vi "Teleop-2022-comp.vi"(10 "Match Info":T1={"Autonomous Elapsed Seconds"=0.0, "TeleOp Elapsed Seconds"=0.0, "Disabled Elapsed Seconds"=0.0, "Visited Autonomous"=FALSE, "Visited TeleOp"=FALSE, "Visited Disabled"=FALSE, "Autonomous Settings"={"Autonomous Style"=enum."Independent", "VI Refnum"=refnum}}, 11 "Call Context":T2) -> ()   [LabVIEW 2020]
doc: "This VI is called for each TeleOp packet received from the DS where the robot is not disabled. It is often used to read from the joysticks and update I/O or to update setpoints for timed control loops. It should complete and return within 20 milliseconds or it may miss DS packets."
uses:
  <vilib>/Rock Robotics/WPI/DriverStation/WPI_DriverStationDerivedRobotMode.ctl
  <vilib>/Rock Robotics/WPI/DriverStation/WPI_DriverStationMatch Info.ctl
  <vilib>/Rock Robotics/WPI/Joystick/XBox Buttons Indexer.ctl
  <vilib>/Rock Robotics/WPI/Joystick/XBox Axes Indexer.ctl
  <vilib>/Rock Robotics/WPI/Relay/WPI_RelayValue.ctl
  <vilib>/Rock Robotics/Network Tables/NT Read Boolean.vi
  <vilib>/Rock Robotics/Network Tables/NT Read Number.vi
  Auxilary/AuxGlobals.vi
  Climb/ClimbGlobals.vi
  <vilib>/Rock Robotics/Network Tables/NT Write String.vi
  Human/HumanGlobal.vi
  DriveSystem/DriveGlobals.vi
  <vilib>/Rock Robotics/Network Tables/NT Write Number.vi
  <vilib>/Rock Robotics/Network Tables/NT Write Boolean.vi
  Vision/VisionGlobals.vi
  <vilib>/Rock Robotics/WPI/Joystick/WPI_JoystickArcadeMapping.vi
  <vilib>/Rock Robotics/WPI/ThirdParty/JAS_Junk/TrajLib/Trajectory_Library.lvlib
panel:
  out "Sample Slider 0":dbl(slide) scale=0.0..5.0
  out "Sample Boolean 1":bool
  out "Sample Boolean 0":bool
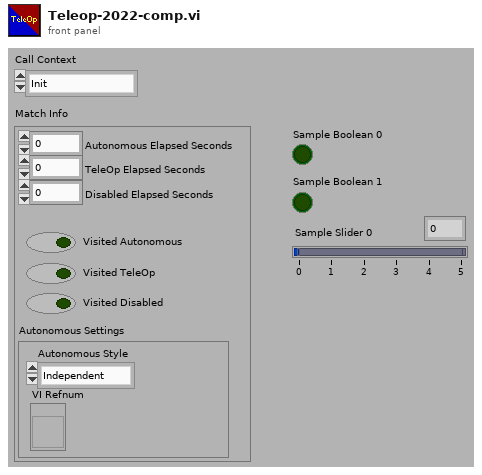
[diagram p1: front panel]
types:
  T1 = typedef "WPI_DriverStationMatch Info.ctl" = cluster{"Autonomous Elapsed Seconds":dbl, "TeleOp Elapsed Seconds":dbl, "Disabled Elapsed Seconds":dbl, "Visited Autonomous":bool, "Visited TeleOp":bool, "Visited Disabled":bool, "Autonomous Settings":cluster{"Autonomous Style":enum16{"Iterative", "Independent"}, "VI Refnum":refnum<vi>}}
  T2 = typedef "WPI_DriverStationDerivedRobotMode.ctl" = enum16{"Init", "Execute", "Stop"}
  T3 = typedef "XBox Buttons Indexer.ctl" = enum16{"A", "B", "X", "Y", "Left Bumper", "Right Bumper", "Back", "Start", "Left Joystick", "Right Joystick"}
  T4 = typedef "XBox Axes Indexer.ctl" = enum16{"Left X", "Left Y", "Left Trigger", "Right Trigger", "Right X", "Right Y"}
  T5 = typedef "WPI_RelayValue.ctl" = enum16{"Off", "On", "Forward", "Reverse"}
  T6 = typedef "WPI_RelayDevRef.ctl" = cluster{"DevStatus":errorcluster, "Relay Channel":T7, "Relay Direction":T8}
  T7 = typedef "FPGA_DIORelayChannel.ctl" = enum8{"Relay 0", "Relay 1", "Relay 2", "Relay 3", "Invalid"}
  T8 = typedef "WPI_RelayDirection.ctl" = enum16{"Both directions", "Forward only", "Reverse only"}
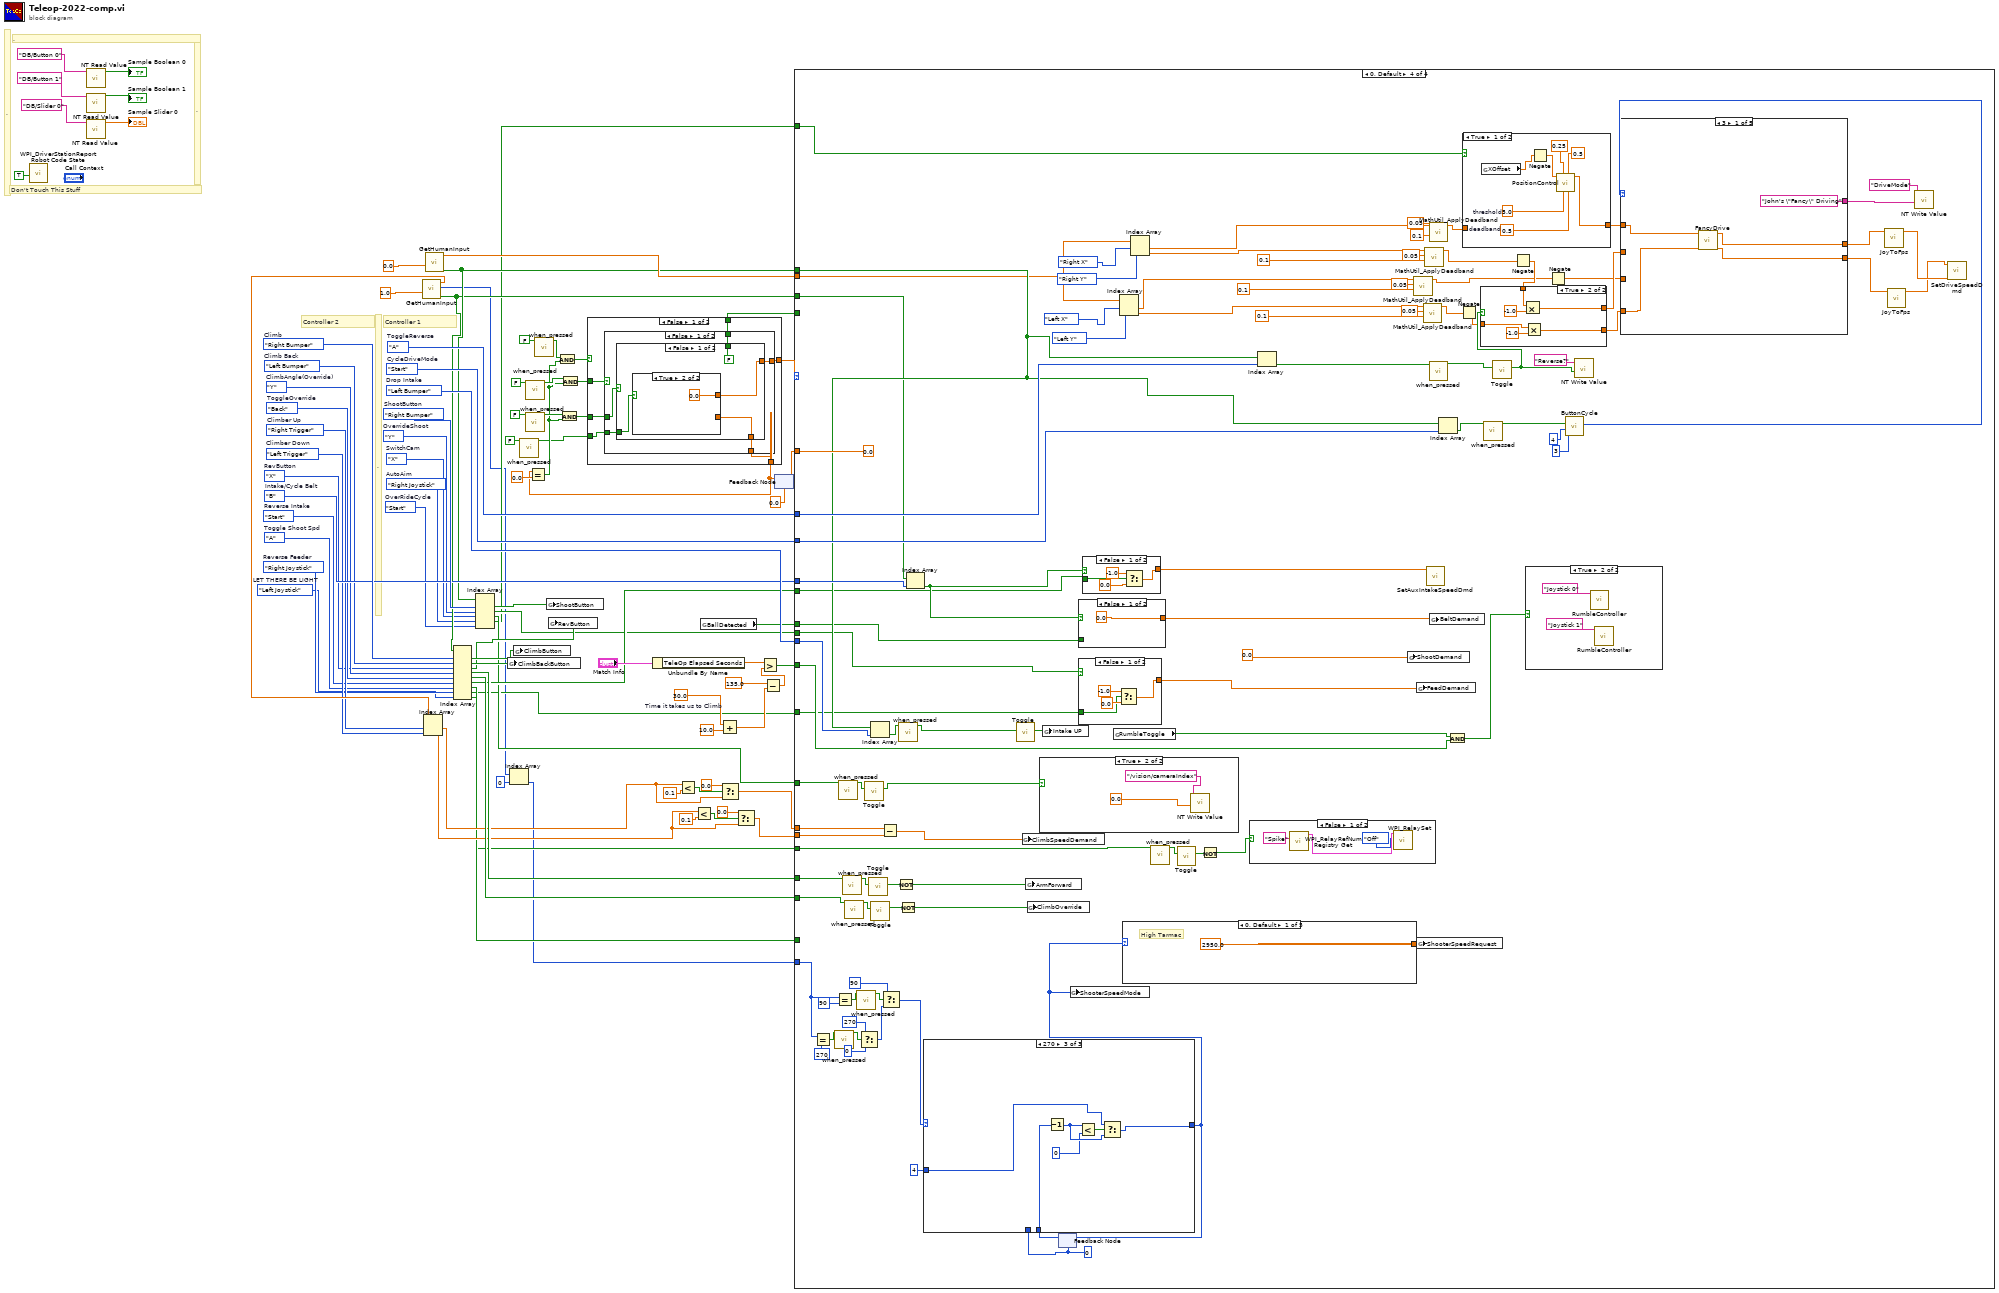
[diagram p0: block diagram]
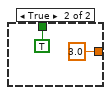
[diagram p3: hidden frame]
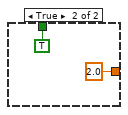
[diagram p4: hidden frame]
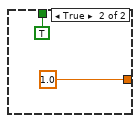
[diagram p5: hidden frame]
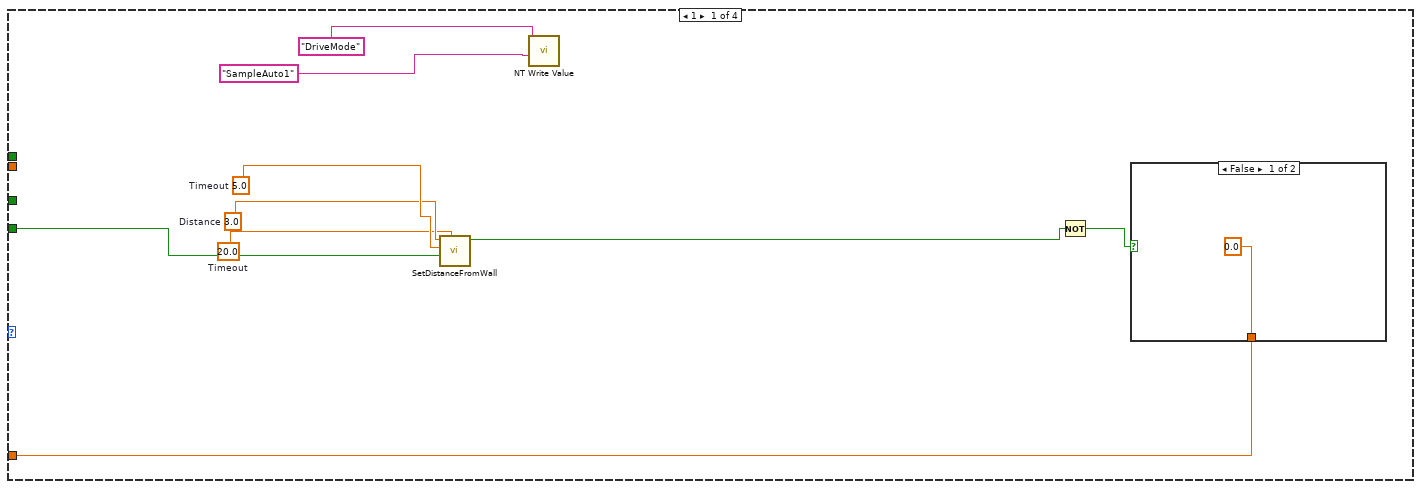
[diagram p6: hidden frame]
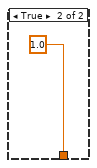
[diagram p7: hidden frame]
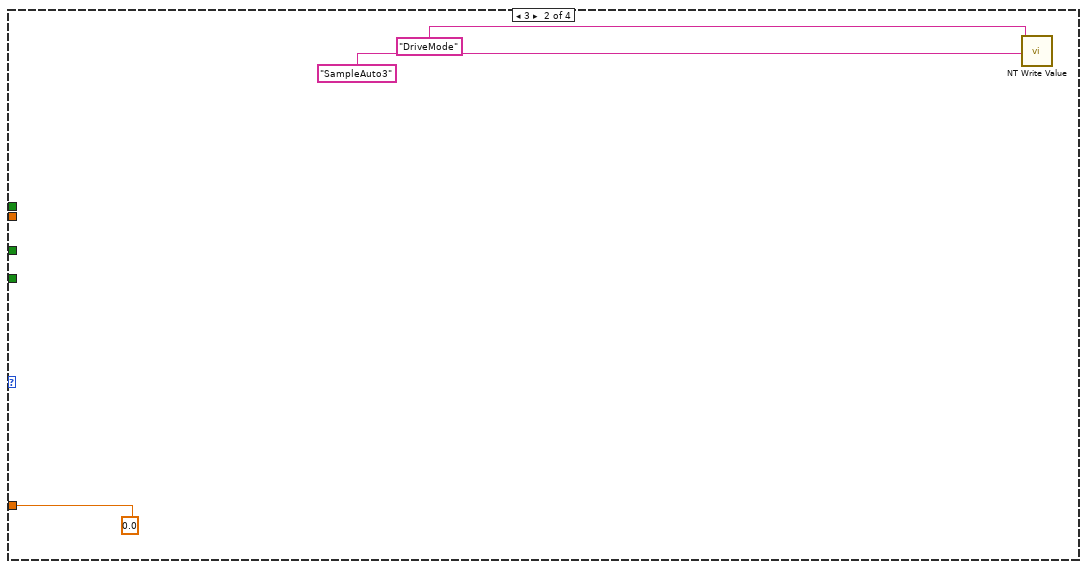
[diagram p8: hidden frame]
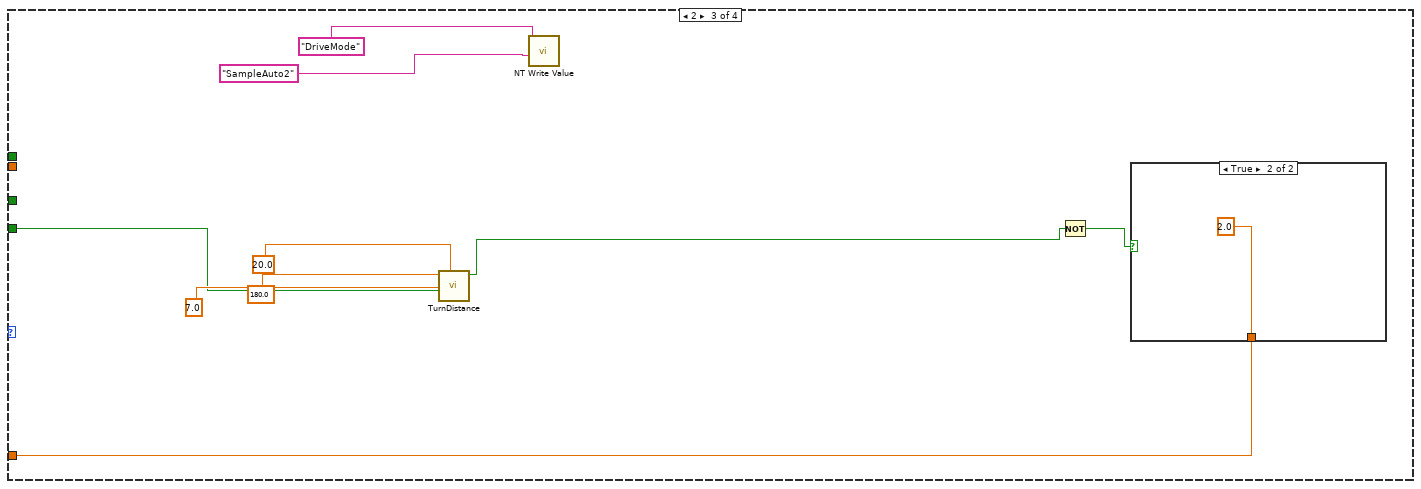
[diagram p9: hidden frame]
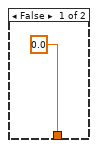
[diagram p10: hidden frame]
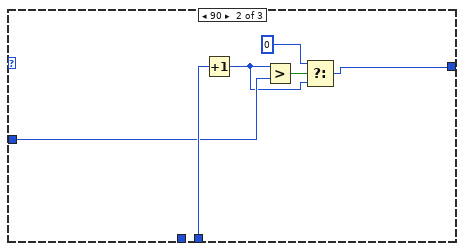
[diagram p12: hidden frame]
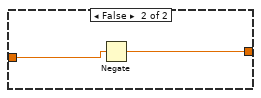
[diagram p13: hidden frame]
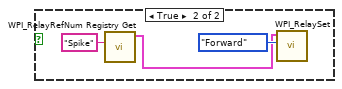
[diagram p14: hidden frame]
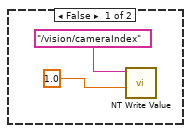
[diagram p15: hidden frame]
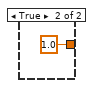
[diagram p16: hidden frame]
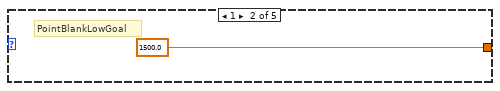
[diagram p17: hidden frame]
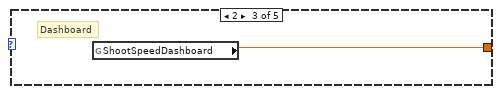
[diagram p18: hidden frame]
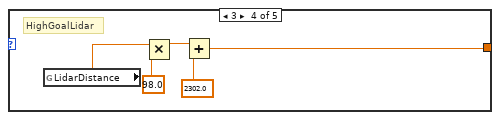
[diagram p19: hidden frame]
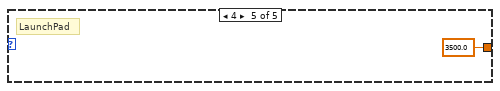
[diagram p20: hidden frame]
diagram:
  w1 = XBox_Buttons_Indexer."Start"  # OverRideCycle
  w6 = XBox_Buttons_Indexer."Right Joystick"  # AutoAim
  w8 = XBox_Buttons_Indexer."Left Joystick"  # LET THERE BE LIGHT
  w10 = XBox_Buttons_Indexer."Right Joystick"  # Reverse Feeder
  w12 = XBox_Buttons_Indexer."X"  # SwitchCam
  w15 = XBox_Buttons_Indexer."Y"  # OverrideShoot
  w17 = XBox_Buttons_Indexer."A"  # Toggle Shoot Spd
  w29 = XBox_Buttons_Indexer."Start"  # Reverse Intake
  w39 = XBox_Buttons_Indexer."Left Bumper"  # Climb Back
  w40 = XBox_Axes_Indexer."Left Trigger"  # Climber Down
  w41 = XBox_Axes_Indexer."Right Trigger"  # Climber Up
  w44 = XBox_Buttons_Indexer."Back"  # ToggleOverride
  w45 = XBox_Buttons_Indexer."Y"  # ClimbAngle(Override)
  w49 = XBox_Buttons_Indexer."Right Bumper"  # Climb
  w51 = XBox_Buttons_Indexer."Left Bumper"  # Drop Intake
  w48 = XBox_Buttons_Indexer."B"  # Intake/Cycle Belt
  w59 = 30.0  # Time it takes us to Climb
  w32 = XBox_Buttons_Indexer."X"  # RevButton
  w53 = XBox_Buttons_Indexer."Right Bumper"  # ShootButton
  w62 = XBox_Buttons_Indexer."Start"  # CycleDriveMode
  w63 = XBox_Buttons_Indexer."A"  # ToggleReverse
  # "."
  # "Controller 2"
  # "Controller 1"
  # "."
  # "."
  # "."
  # "Don't Touch This Stuff"
  n1 = call <vilib>:"WPI_DriverStationReport Robot Code State.vi"("TeleOp"=TRUE ("Autonomous")) -> ()  [unwired: 10 in, 1 out]
  n2 = call-poly <vilib>:"NT Read Value.vi"("name"="DB/Button 0" ("refnum name")) -> ("value"=→"Sample Boolean 0":bool)  [unwired: 8 in, 2 out]
  n3 = call-poly <vilib>:"NT Read Value.vi"("name"="DB/Slider 0" ("refnum name")) -> ("value"=→"Sample Slider 0":dbl)  [unwired: 8 in, 2 out]
  n4 = call-poly <vilib>:"NT Read Value.vi"("name"="DB/Button 1" ("refnum name")) -> ("value"=→"Sample Boolean 1":bool)  [unwired: 8 in, 2 out]
  n5 = call "GetHumanInput.vi"("Controller"=1.0) -> ("Buttons"=w30:bool[], "POVs"=w4:i16[], "Axes"=w42:dbl[])  [unwired: 8 in]
  n6 = Index Array(array=w42, index #1=w41, index #2=w40) -> (element #1=w25:dbl, element #2=w19:dbl)
  n7 = call "GetHumanInput.vi"("Controller"=0.0) -> ("Buttons"=w37:bool[], "Axes"=w78:dbl[])  [unwired: 8 in, 1 out]
  n8 = Index Array(array=w30, index #1=w49, index #2=w39, index #3=w32, index #4=w45, index #5=w44, index #6=w29, index #7=w17, index #8=w10, index #9=w8) -> (element #1=w50:bool, element #2=w38:bool, element #3=w31:bool, element #4=w46:bool, element #5=w43:bool, element #6=w28:bool, element #7=w16:bool, element #8=w9:bool, element #9=w7:bool)
  n9 = Index Array(array=w37, index #1=w53, index #2=w15, index #3=w12, index #4=w6, index #5=w1) -> (element #1=w54:bool, element #2=w14:bool, element #3=w11:bool, element #4=w5:bool)  [unwired: 1 out]
  n10 = global write "ClimbGlobals.vi" "ClimbBackButton"(w38) -> ()
  n11 = Index Array(array=w4, index=0) -> (element=w2:i16)
  n12 = global write "ClimbGlobals.vi" "ClimbButton"(w50) -> ()
  n13 = call "when_pressed.vi"("Input"=FALSE) -> ("Output"=w64:bool)  [unwired: 10 in]
  n14 = call "when_pressed.vi"("Input"=FALSE) -> ("Output"=w68:bool)  [unwired: 10 in]
  n15 = call "when_pressed.vi"("Input"=FALSE) -> ("Output"=w67:bool)  [unwired: 10 in]
  n16 = call "when_pressed.vi"("Input"=FALSE) -> ("Output"=w71:bool)  [unwired: 10 in]
  n17 = global write "AuxGlobals.vi" "ShootButton"(w54) -> ()
  n18 = global write "AuxGlobals.vi" "RevButton"(w31) -> ()
  n19 = Unbundle By Name("Match Info") -> ("TeleOp Elapsed Seconds"=w61:dbl)
  n20 = Less?(x=w25, y=0.1) -> (x < y?=w26:bool)
  n21 = Less?(x=w19, y=0.1) -> (x < y?=w21:bool)
  n22 = global read "AuxGlobals.vi" "BallDetected"() -> (w47:bool)
  n23 = Add(x=w59, y=10.0) -> (x+y=w57:dbl)
  n24 = Select(t=0.0, s=w26, f=w25) -> (s? t:f=w23:dbl)
  n25 = Select(t=0.0, s=w21, f=w19) -> (s? t:f=w18:dbl)
  n26 = Subtract(x=135.0 ("y"), y=w57) -> (x-y=w56:dbl)
  n27 = Greater?(x=w61, y=w56) -> (0:w55:bool)
  n28 = feedback #1(0.0) -> (w73:dbl)
  n29 = Equal?(x=w73, y=0.0) -> (x = y?=w66:bool)
  n30 = And(x=w71, y=w66) -> (x .and. y?=w72:bool)
  n31 = And(x=w68, y=w66) -> (x .and. y?=w69:bool)
  n32 = And(x=w67, y=w66) -> (x .and. y?=w70:bool)
  n33 = case shown="False" w72 {
    tunnel: [w89 1.0] -> w13
    tunnel: w73 -> [w90 _]
    tunnel: w70 -> [w92 _]
    tunnel: w69 -> [w91 _]
    tunnel: [w88 TRUE] -> w65
    tunnel: w64 -> [w87 _]
    frame False {
      n34 = case shown="False" w92 {
        tunnel: w91 -> [w97 _]
        tunnel: w90 -> [w96 _]
        tunnel: [w95 2.0] -> w89
        tunnel: [w94 TRUE] -> w88
        tunnel: w87 -> [w93 _]
        frame False {
          n35 = case shown="False" w97 {
            tunnel: w96 -> [w98 _]
            tunnel: [w99 3.0] -> w95
            tunnel: [FALSE TRUE] -> w94
            tunnel: w93 -> [w100 _]
            frame False {
              n36 = case shown="True" w100 {
                tunnel: [w102 0.0] -> w99
                tunnel: w98 -> [w102 _]
                frame False {
                }
                frame True {
                }
              }
            }
            frame True {
            }
          }
        }
        frame True {
        }
      }
    }
    frame True {
    }
  }
  n37 = case shown="0, Default" w13 {
    tunnel: w78 -> [_ _ _ w183]
    tunnel: w37 -> [_ _ _ w201]
    tunnel: [w111 0.0 w129 0.0] -> w76
    tunnel: w65 -> [w110 _ w124 _]
    tunnel: w63 -> [_ _ _ w209]
    tunnel: w62 -> [_ _ _ w208]
    tunnel: w55 -> [_ _ _ w204]
    tunnel: w48 -> [_ _ _ w206]
    tunnel: w51 -> [_ _ _ w200]
    tunnel: w47 -> [_ _ _ w181]
    tunnel: w46 -> [_ _ _ w177]
    tunnel: w43 -> [_ _ _ w175]
    tunnel: w23 -> [_ _ _ w174]
    tunnel: w18 -> [_ _ _ w173]
    tunnel: w30 -> [_ _ _ w172]
    tunnel: w28 -> [_ _ _ w171]
    tunnel: w16 -> [_ _ _ _]
    tunnel: w14 -> [_ _ _ w164]
    tunnel: w11 -> [_ _ _ w161]
    tunnel: w9 -> [_ _ _ w160]
    tunnel: w7 -> [_ _ _ w156]
    tunnel: w5 -> [_ _ _ w155]
    tunnel: w2 -> [_ _ _ w140]
    frame 1 {
      w114 = 20.0  # Timeout
      w115 = 3.0  # Distance
      w116 = 5.0  # Timeout
      n38 = call "SetDistanceFromWall.vi"("Timeout"=w114, "Initation?"=w110, "MaxSpeed"=w116, "Distance"=w115) -> ("Finished"=w113:bool)  [unwired: 5 in, 2 out]
      n39 = call-poly <vilib>:"NT Write Value.vi"("value"="SampleAuto1" ("String"), "name"="DriveMode" ("Name")) -> ()  [unwired: 9 in, 1 out]
      n40 = Not(x=w113) -> (.not. x?=w112:bool)
      n41 = case shown="False" w112 {
        tunnel: [0.0 1.0] -> w111
        frame False {
        }
        frame True {
        }
      }
    }
    frame 3 {
      n42 = call-poly <vilib>:"NT Write Value.vi"("value"="SampleAuto3" ("String"), "name"="DriveMode" ("Name")) -> ()  [unwired: 9 in, 1 out]
    }
    frame 2 {
      n43 = call "TurnDistance.vi"("Timeout"=20.0, "Initation?"=w124, "MaxSpeed"=7.0, "Degrees"=180.0) -> ("Finished"=w128:bool)  [unwired: 5 in, 2 out]
      n44 = call-poly <vilib>:"NT Write Value.vi"("value"="SampleAuto2" ("String"), "name"="DriveMode" ("Name")) -> ()  [unwired: 9 in, 1 out]
      n45 = Not(x=w128) -> (.not. x?=w130:bool)
      n46 = case shown="True" w130 {
        tunnel: [0.0 2.0] -> w129
        frame False {
        }
        frame True {
        }
      }
    }
    frame 0, Default {
      w153 = 0
      n47 = Equal?(x=w140, y=i16 270) -> (x = y?=w147:bool)
      n48 = call "when_pressed.vi"("Input"=w147) -> ("Output"=w146:bool)  [unwired: 10 in]
      n49 = Equal?(x=w140, y=i16 90) -> (x = y?=w150:bool)
      n50 = call "when_pressed.vi"("Input"=w161) -> ("Output"=w163:bool)  [unwired: 10 in]
      n51 = call "when_pressed.vi"("Input"=w177) -> ("Output"=w178:bool)  [unwired: 10 in]
      n52 = call "when_pressed.vi"("Input"=w175) -> ("Output"=w176:bool)  [unwired: 10 in]
      n53 = call "when_pressed.vi"("Input"=w150) -> ("Output"=w149:bool)  [unwired: 10 in]
      n54 = Select(t=270, s=w146, f=0) -> (s? t:f=w142:i32)
      n55 = call "Toggle.vi"("FlashInput"=w163) -> ("On/Off"=w162:bool)  [unwired: 10 in]
      n56 = call "Toggle.vi"("FlashInput"=w178) -> ("On/Off"=w170:bool)  [unwired: 10 in]
      n57 = call "Toggle.vi"("FlashInput"=w176) -> ("On/Off"=w167:bool)  [unwired: 10 in]
      n58 = Index Array(array=w201, index=w200) -> (element=w198:bool)
      n59 = Subtract(x=w174, y=w173) -> (x-y=w182:dbl)
      n60 = Select(t=90, s=w149, f=w142) -> (s? t:f=w139:i32)
      n61 = Not(x=w170) -> (.not. x?=w169:bool)
      n62 = call "when_pressed.vi"("Input"=w198) -> ("Output"=w199:bool)  [unwired: 10 in]
      n63 = Not(x=w167) -> (.not. x?=w168:bool)
      n64 = Index Array(array=w172, index=w206) -> (element=w180:bool)
      n65 = call "Toggle.vi"("FlashInput"=w199) -> ("On/Off"=w202:bool)  [unwired: 10 in]
      n66 = global write "ClimbGlobals.vi" "ClimbSpeedDemand"(w182) -> ()
      n67 = global write "ClimbGlobals.vi" "ArmForward"(w169) -> ()
      n68 = global write "ClimbGlobals.vi" "ClimbOverride"(w168) -> ()
      n69 = case shown="True" w162 {
        frame False {
          n70 = call-poly <vilib>:"NT Write Value.vi"("value"=1.0, "name"="/vision/cameraIndex" ("Name")) -> ()  [unwired: 9 in, 1 out]
        }
        frame True {
          n71 = call-poly <vilib>:"NT Write Value.vi"("value"=0.0, "name"="/vision/cameraIndex" ("Name")) -> ()  [unwired: 9 in, 1 out]
        }
      }
      n72 = global write "AuxGlobals.vi" "Intake UP"(w202) -> ()
      n73 = feedback #2(w153) -> (w154:i32)
      n74 = case shown="270" w139 {
        tunnel: [w235 w236 w246] -> w151
        tunnel: w154 -> [w235 w241 w244]
        tunnel: w153 -> [_ _ _]
        tunnel: 4 ("MaxNum") -> [_ w239 w243]
        frame 0, Default {
        }
        frame 90 {
          n75 = Increment(x=w241) -> (x+1=w237:i32)
          n76 = Greater?(x=w237, y=w239) -> (0:w240:bool)
          n77 = Select(t=0, s=w240, f=w237) -> (s? t:f=w236:i32)
        }
        frame 270 {
          n78 = Decrement(x=w244) -> (x-1=w245:i32)
          n79 = Less?(x=w245, y=0) -> (x < y?=w247:bool)
          n80 = Select(t=w243, s=w247, f=w245) -> (s? t:f=w246:i32)
        }
      }
      n81 = feedback-in #2(w151) -> ()
      n82 = global write "AuxGlobals.vi" "ShooterSpeedMode"(w151) -> ()
      n83 = case shown="False" w180 {
        tunnel: [0.0 ("Shooter Demand") w284] -> w197
        tunnel: w181 -> [_ w282]
        frame False {
        }
        frame True {
          n84 = Select(t=0.0 ("Shooter Demand"), s=w282, f=0.8) -> (s? t:f=w284:dbl)
        }
      }
      n85 = case shown="False" w164 {
        tunnel: [w267 1.0 ("FeedDemand")] -> w165
        tunnel: w160 -> [w268 _]
        frame False {
          n86 = Select(t=-1.0, s=w268, f=0.0 ("FeedDemand")) -> (s? t:f=w267:dbl)
        }
        frame True {
        }
      }
      n87 = case shown="False" w180 {
        tunnel: [w286 1.0 ("Shooter Demand")] -> w207
        tunnel: w171 -> [w287 _]
        frame False {
          n88 = Select(t=-1.0, s=w287, f=0.0 ("Shooter Demand")) -> (s? t:f=w286:dbl)
        }
        frame True {
        }
      }
      n89 = global read "HumanGlobal.vi" "RumbleToggle"() -> (w205:bool)
      n90 = Index Array(array=w183, index #1=XBox_Axes_Indexer."Left X" ("XBox Axes"), index #2=XBox_Axes_Indexer."Left Y" ("XBox Axes")) -> (element #1=w187:dbl, element #2=w184:dbl)
      n91 = case shown="0, Default" w151 {
        tunnel: [2950.0 ("ShootSpeedDashboard") 1500.0 ("ShootSpeedDashboard") w274 w275 3500.0 ("ShootSpeedDashboard")] -> w166
        frame 0, Default {
          # "High Tarmac"
        }
        frame 1 {
          # "PointBlankLowGoal"
        }
        frame 2 {
          # "Dashboard"
          n92 = global read "AuxGlobals.vi" "ShootSpeedDashboard"() -> (w274:dbl)
        }
        frame 3 {
          # "HighGoalLidar"
          n93 = global read "DriveGlobals.vi" "LidarDistance"() -> (w279:dbl)
          n94 = Multiply(x=w279, y=98.0) -> (x*y=w277:dbl)
          n95 = Add(x=w277, y=2302.0) -> (x+y=w275:dbl)
        }
        frame 4 {
          # "LaunchPad"
        }
      }
      n96 = Index Array(array=w183, index #1=XBox_Axes_Indexer."Right X" ("XBox Axes"), index #2=XBox_Axes_Indexer."Right Y" ("XBox Axes")) -> (element #1=w193:dbl, element #2=w190:dbl)
      n97 = call "when_pressed.vi"("Input"=w156) -> ("Output"=w159:bool)  [unwired: 10 in]
      n98 = call "Toggle.vi"("FlashInput"=w159) -> ("On/Off"=w158:bool)  [unwired: 10 in]
      n99 = Not(x=w158) -> (.not. x?=w157:bool)
      n100 = case shown="False" w157 {
        frame False {
          n101 = call <vilib>:"WPI_RelayRefNum Registry Get.vi"("refnum name"="Spike") -> ("RelayDevRef"=w259:T6)  [unwired: 9 in, 1 out]
          n102 = call <vilib>:"WPI_RelaySet.vi"("RelayValue"=WPI_RelayValue."Off", "RelayDevRef"=w259) -> ()  [unwired: 8 in, 2 out]
        }
        frame True {
          n103 = call <vilib>:"WPI_RelayRefNum Registry Get.vi"("refnum name"="Spike") -> ("RelayDevRef"=w260:T6)  [unwired: 9 in, 1 out]
          n104 = call <vilib>:"WPI_RelaySet.vi"("RelayValue"=WPI_RelayValue."Forward", "RelayDevRef"=w260) -> ()  [unwired: 8 in, 2 out]
        }
      }
      n105 = Index Array(array=w201, index=w209) -> (element=w227:bool)
      n106 = global write "AuxGlobals.vi" "ShootDemand"(0.0 ("ShootDemand")) -> ()
      n107 = call <vilib>:"MathUtil_ApplyDeadband.vi"("Max Magnitude"=0.1 ("Deadband"), "Deadband"=0.05, "Value"=w187) -> ("Result"=w188:dbl)  [unwired: 8 in]
      n108 = global write "AuxGlobals.vi" "FeedDemand"(w165) -> ()
      n109 = global write "AuxGlobals.vi" "ShooterSpeedRequest"(w166) -> ()
      n110 = call <vilib>:"MathUtil_ApplyDeadband.vi"("Max Magnitude"=0.1 ("Deadband"), "Deadband"=0.05, "Value"=w184) -> ("Result"=w185:dbl)  [unwired: 8 in]
      n111 = call <vilib>:"MathUtil_ApplyDeadband.vi"("Max Magnitude"=0.1 ("Deadband"), "Deadband"=0.05, "Value"=w190) -> ("Result"=w191:dbl)  [unwired: 8 in]
      n112 = call "SetAuxIntakeSpeedDmd.vi"("IntakeDemand"=w207) -> ()  [unwired: 11 in]
      n113 = call <vilib>:"MathUtil_ApplyDeadband.vi"("Max Magnitude"=0.1 ("Deadband"), "Deadband"=0.05, "Value"=w193) -> ("Result"=w194:dbl)  [unwired: 8 in]
      n114 = call "when_pressed.vi"("Input"=w227) -> ("Output"=w225:bool)  [unwired: 10 in]
      n115 = global write "AuxGlobals.vi" "BeltDemand"(w197) -> ()
      n116 = Index Array(array=w201, index=w208) -> (element=w233:bool)
      n117 = And(x=w205, y=w204) -> (x .and. y?=w203:bool)
      n118 = Negate(x=w185) -> (-x=w218:dbl)
      n119 = case shown="True" w155 {
        tunnel: [w254 w256] -> w221
        tunnel: w194 -> [_ w255]
        frame True {
          w250 = 5.0  # threshold
          w251 = 0.5  # deadband
          n120 = global read "VisionGlobals.vi" "XOffset"() -> (w249:dbl)
          n121 = Negate(x=w249) -> (-x=w248:dbl)
          n122 = call "PositionControl.vi"("deadband"=w251, "maxdemand"=0.5, "threshold"=w250, "mindemand"=0.25, "Error"=w248) -> ("output variable"=w254:dbl)  [unwired: 5 in, 1 out]
        }
        frame False {
          n123 = Negate(x=w255) -> (-x=w256:dbl)
        }
      }
      n124 = call "when_pressed.vi"("Input"=w233) -> ("Output"=w217:bool)  [unwired: 10 in]
      n125 = call "Toggle.vi"("FlashInput"=w225) -> ("On/Off"=w223:bool)  [unwired: 10 in]
      n126 = Negate(x=w191) -> (-x=w220:dbl)
      n127 = case shown="True" w223 {
        tunnel: w220 -> [w295 w300]
        tunnel: w218 -> [w294 w298]
        tunnel: [w294 w297] -> w224
        tunnel: [w295 w296] -> w222
        frame False {
        }
        frame True {
          n128 = Multiply(x=w300, y=-1.0) -> (x*y=w296:dbl)
          n129 = Multiply(x=w298, y=-1.0) -> (x*y=w297:dbl)
        }
      }
      n130 = case shown="True" w203 {
        frame False {
          n131 = call "StopRumble.vi"("Controller Name"="Joystick 0") -> ()  [unwired: 11 in]
        }
        frame True {
          n132 = call "RumbleController.vi"("Controller Name"="Joystick 0") -> ()  [unwired: 11 in]
          n133 = call "RumbleController.vi"("Controller Name"="Joystick 1") -> ()  [unwired: 11 in]
        }
      }
      n134 = Negate(x=w188) -> (-x=w219:dbl)
      n135 = call "ButtonCycle.vi"("Start At"=3, "MaxNum"=4, "FlashInput"=w217) -> ("CycleNumber"=w216:i32)  [unwired: 8 in]
      n136 = call-poly <vilib>:"NT Write Value.vi"("value"=w223, "name"="Reverse?" ("Name")) -> ()  [unwired: 9 in, 1 out]
      n137 = case shown="3" w216 {
        tunnel: w219 -> [_ _ _ w325 _]
        tunnel: w224 -> [w304 w309 w319 w324 w326]
        tunnel: [w302 w310 w313 w323 w326] -> w232
        tunnel: [w303 w311 w312 w322 w327] -> w231
        tunnel: w221 -> [w305 w308 w320 _ _]
        tunnel: ["John's \"Fancy\" Driving" "Dual Arcade" "Precision" "Arcade" "Tank"] -> w228
        tunnel: w222 -> [_ _ _ _ w327]
        frame 3 {
          n138 = call "FancyDrive.vi"("Y axis value"=w304, "X axis value"=w305) -> ("Right Motor Value"=w303:dbl, "Left Motor Value"=w302:dbl)  [unwired: 8 in]
        }
        frame 1 {
          n139 = call-poly <vilib>:"WPI_JoystickMapping.vi"("Y axis value"=w309, "X axis value"=w308) -> ("Right Motor Value"=w311:dbl, "Left Motor Value"=w310:dbl)  [unwired: 8 in]
        }
        frame 2 {
          n140 = call-poly <vilib>:"WPI_JoystickMapping.vi"("Y axis value"=w319, "X axis value"=w320) -> ("Right Motor Value"=w317:dbl, "Left Motor Value"=w316:dbl)  [unwired: 8 in]
          n141 = Multiply(x=w316, y=0.5) -> (x*y=w313:dbl)
          n142 = Multiply(x=w317, y=0.5) -> (x*y=w312:dbl)
        }
        frame 0, Default {
          n143 = call-poly <vilib>:"WPI_JoystickMapping.vi"("Y axis value"=w324, "X axis value"=w325) -> ("Right Motor Value"=w322:dbl, "Left Motor Value"=w323:dbl)  [unwired: 8 in]
        }
        frame 4 {
        }
      }
      n144 = call "JoyToFps.vi"("JoystickInput"=w232) -> ("Fps"=w230:dbl)  [unwired: 10 in]
      n145 = call "JoyToFps.vi"("JoystickInput"=w231) -> ("Fps"=w229:dbl)  [unwired: 10 in]
      n146 = call-poly <vilib>:"NT Write Value.vi"("value"=w228, "name"="DriveMode" ("Name")) -> ()  [unwired: 9 in, 1 out]
      n147 = call "SetDriveSpeedDmd.vi"("LeftSpeedInput"=w230, "RightSpeedInput"=w229) -> ()  [unwired: 10 in]
    }
  }
  n148 = feedback-in #1(w76) -> ()
